vi "Wait-for-execution-end.vi"(8 "error in (no error)":errorcluster, 11 "VI in":refnum<vi>) -> (0 "error out":errorcluster, 3 "VI out":refnum<vi>)   [LabVIEW 2013, in "PowderDeposition.lvlib" / "Motor-assembly.lvclass"]
uses:
  Motor-assembly.lvclass
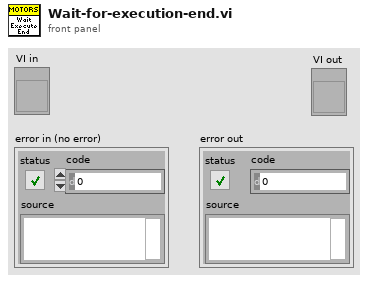
[diagram p1: front panel]
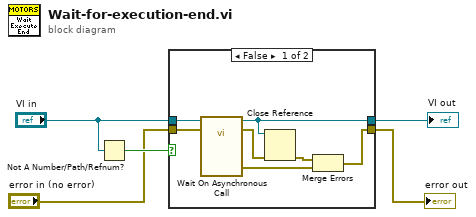
[diagram p0: block diagram]
diagram:
  n1 = Not A Number/Path/Refnum?(number/path/refnum="VI in") -> (NaN/Path/Refnum?=w3:bool)
  n2 = case shown="False" w3 {
    tunnel: "VI in" -> [w12 w13]
    tunnel: "error in (no error)" -> [w11 w14]
    tunnel: [w7 w14] -> w5
    tunnel: [w6 w13] -> w1
    frame False {
      n3 = call-by-ref "Wait On Asynchronous Call"(reference=w12, error in=w11) -> (reference out=w6:refnum<vi>, error out=w10:errorcluster, 0:"error out"=w8:errorcluster)  [unwired: 10 in, 1 out]
      n4 = Close Reference(reference=w6, error in (no error)=w10) -> (error out=w9:errorcluster)
      n5 = Merge Errors(w9, w8) -> (w7:errorcluster)
    }
    frame True {
    }
  }
  "error out" <- w5
  "VI out" <- w1
